vi "SwerveKinematics_NormalizeWheelSpeedsX.vi"(9 "AttainableMaxSpeed":dbl, 11 "in WheelStates":T1[](array[typedef]) {"Angle"."SIN" format="%13.4f"; "Angle"."COS" format="%13.4f"; "Angle"."VALUE" format="%13.4f"}) -> (3 "out WheelStates":T1[](array[typedef]) {"Angle"."SIN" format="%13.4f"; "Angle"."COS" format="%13.4f"; "Angle"."VALUE" format="%13.4f"})   [LabVIEW 2019, in "Trajectory_Library.lvlib"]
doc: "Normalizes the wheel speeds using some max attainable speed. Sometimes, after inverse kinematics, the requested speed from a/several modules may be above the max attainable speed for the driving motor on that module. To fix this issue, one can \"normalize\" all the wheel speeds to make sure that all requested module speeds are below the absolute threshold, while maintaining the ratio of speeds between modules.\n \nParameters:\n - moduleStates - Array of module states. \n - attainableMaxSpeed - The absolute max speed that a module can reach. (Meters/Sec)\n \n\nReturns:\n - out Wheel States -- Array of normalzied Wheel States"
uses:
  Trajectory_Library.lvlib
  TypeDef/ROTATION2D.ctl
  TypeDef/SWERVE_DRIVE_MODULE_STATE.ctl
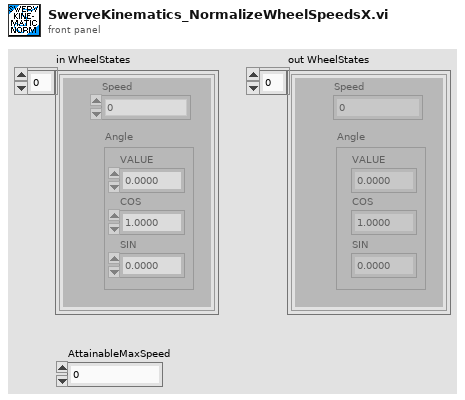
[diagram p1: front panel]
types:
  T1 = typedef "Trajectory_Library.lvlib/SWERVE_DRIVE_MODULE_STATE.ctl" = cluster{"Speed":dbl, "Angle":T2}
  T2 = typedef "Trajectory_Library.lvlib/ROTATION2D.ctl" = cluster{"VALUE":dbl, "COS":dbl, "SIN":dbl}
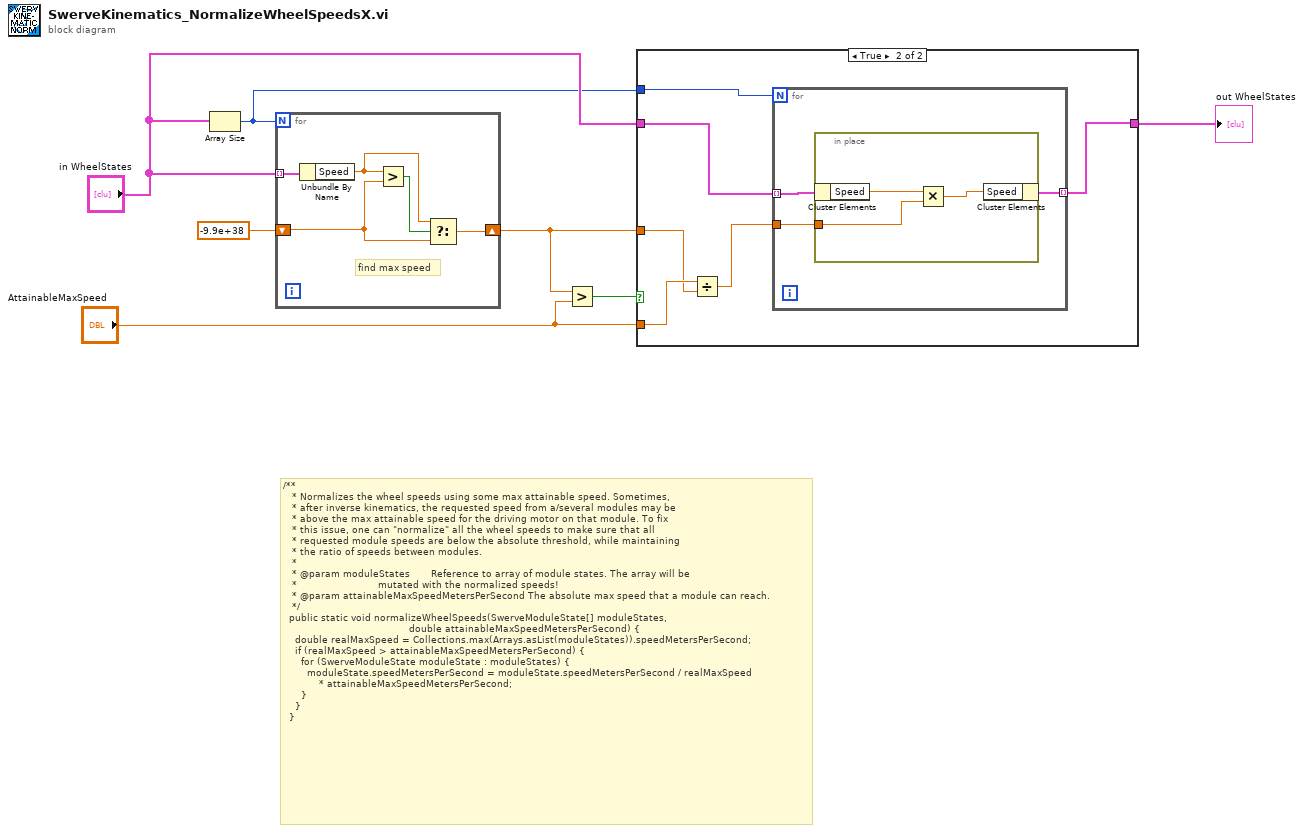
[diagram p0: block diagram]
diagram:
  # "/**\n   * Normalizes the wheel speeds using some max attainable speed. Sometimes,\n   * after inverse kinematics, the requested speed from a/several modules may be\n   * above the max attainable speed for the driving motor on that module. To fix\n   * this issue, one can \"normalize\" all the wheel speeds to make sure that all\n   * requested module speeds are below the absolute threshold, while maintaining\n   * the ratio of speeds between modules.\n   *\n   * @param moduleStates       Reference to array of module states. The array will be\n   *                           mutated with the normalized speeds!\n   * @param attainableMaxSpeedMetersPerSecond The absolute max speed that a module can reach.\n   */\n  public static void normalizeWheelSpeeds(SwerveModuleState[] moduleStates,\n                                          double attainableMaxSpeedMetersPerSecond) {\n    double realMaxSpeed = Collections.max(Arrays.asList(moduleStates)).speedMetersPerSecond;\n    if (realMaxSpeed > attainableMaxSpeedMetersPerSecond) {\n      for (SwerveModuleState moduleState : moduleStates) {\n        moduleState.speedMetersPerSecond = moduleState.speedMetersPerSecond / realMaxSpeed\n            * attainableMaxSpeedMetersPerSecond;\n      }\n    }\n  }"
  n1 = Array Size(array="in WheelStates") -> (size(s)=w1:i32)
  n2 = for {
    N: w1 -> [_]
    shift-right: [w12] -> w2
    shift-left: -9.9e+38 -> [w10]
    tunnel: "in WheelStates" -> [w11] mode=indexing
    # "find max speed"
    n3 = Unbundle By Name(w11) -> ("Speed"=w8:dbl)
    n4 = Greater?(x=w8, y=w10) -> (0:w9:bool)
    n5 = Select(t=w8, s=w9, f=w10) -> (s? t:f=w12:dbl)
  }
  n6 = Greater?(x=w2, y="AttainableMaxSpeed") -> (0:w6:bool)
  n7 = case shown="True" w6 {
    tunnel: "in WheelStates" -> [w13 w17]
    tunnel: [w13 w14] -> w4
    tunnel: "AttainableMaxSpeed" -> [_ w19]
    tunnel: w2 -> [_ w18]
    tunnel: w1 -> [_ w16]
    frame False {
    }
    frame True {
      n8 = Divide(x=w19, y=w18) -> (x/y=w15:dbl)
      n9 = for {
        N: w16 -> [_]
        tunnel: w17 -> [w22] mode=indexing
        tunnel: w15 -> [w21]
        tunnel: [w20] -> w14 mode=indexing
        n10 = in-place {
          in-place-border: w21 -> [w23]
          n11 = in-place-cluster #1(w22) -> ("Speed"=w25:dbl)
          n12 = Multiply(x=w25, y=w23) -> (x*y=w24:dbl)
          n13 = in-place-cluster #1("Speed"=w24) -> (w20:T1)
        }
      }
    }
  }
  "out WheelStates" <- w4
